vi "check Channel to read.vi"() -> ()   [LabVIEW 2019]
uses:
  Controls/Station - Test Type.ctl
  Controls/Global - Device.vi
  Controls/Global - IP Address.vi
  Controls/Global - Device Type.vi
panel:
  out "Array":i32[](array[numeric])
  out "Control Device":i32[](array[numeric])
  out "Device ID":i32[](array[numeric])
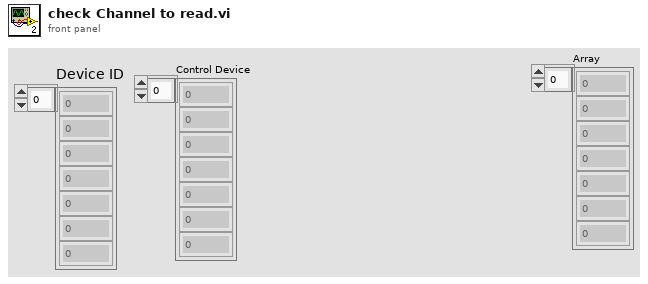
[diagram p1: front panel]
types:
  T1 = typedef "Station - Test Type.ctl" = u16
  T2 = cluster{"Station Name":string, "Key Value":string[], "Key Names":string[]}[]
  T3 = cluster{"Station Name":string, "Key Value":string[], "Key Names":string[]}
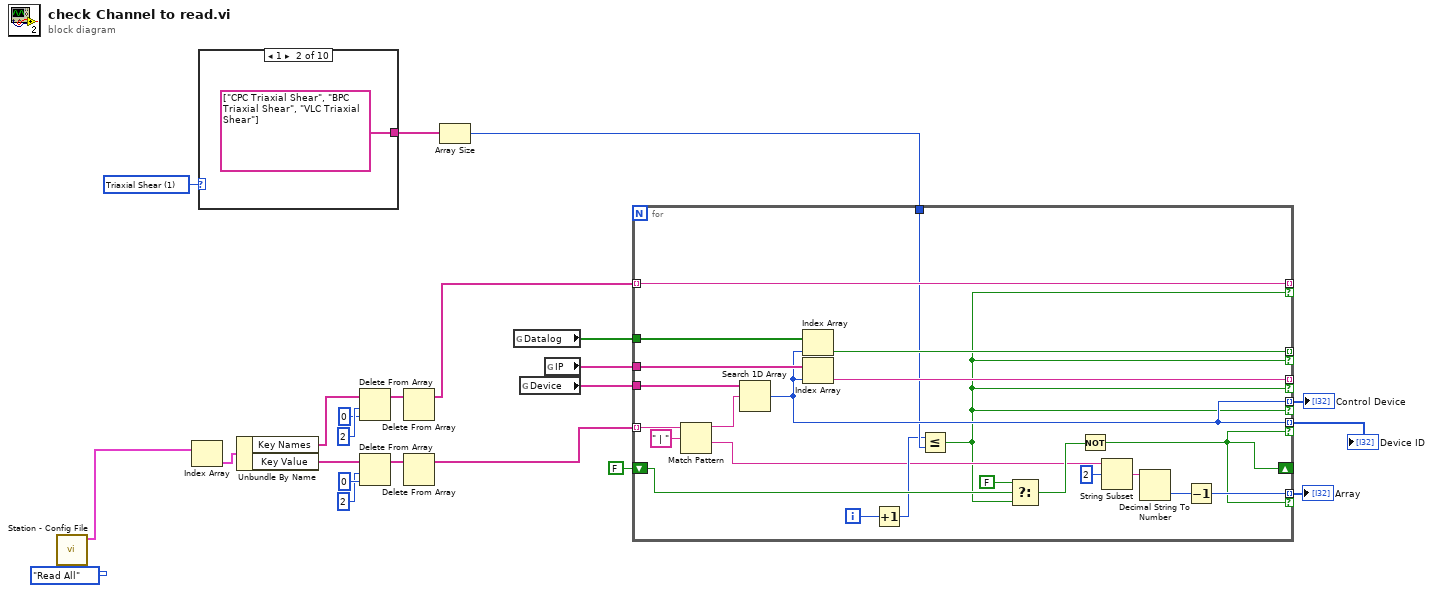
[diagram p0: block diagram]
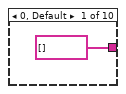
[diagram p2: hidden frame]
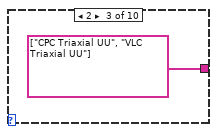
[diagram p3: hidden frame]
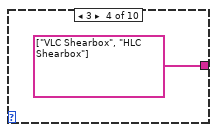
[diagram p4: hidden frame]
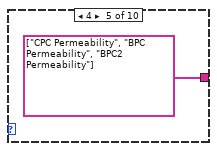
[diagram p5: hidden frame]
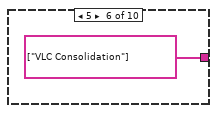
[diagram p6: hidden frame]
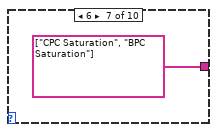
[diagram p7: hidden frame]
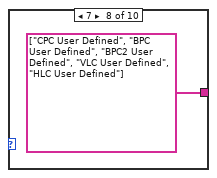
[diagram p8: hidden frame]
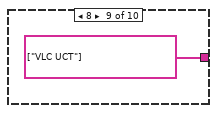
[diagram p9: hidden frame]
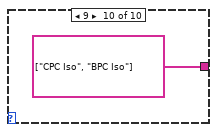
[diagram p10: hidden frame]
diagram:
  w3 = T1 1 items=["Please Select", "Triaxial Shear", "Triaxial UU", "Shearbox", "Permeability", "Consolidation (Stepped Loading)/Swelling", "Saturation (Incremental)", "User Defined", "UCT", "Isotropic Consolidation"] ("Test Type")
  n1 = call "Station - Config File.vi"("Action"=enum16{"Write", "Read", "Read All", "Remove"}."Read All") -> ("Value Out"=w17:T2)  [unwired: 9 in, 1 out]
  n2 = Index Array(array=w17) -> (element=w23:T3)  [unwired: 1 in]
  n3 = case shown="1" w3 {
    tunnel: [string[] [] string[] ["CPC Triaxial Shear", "BPC Triaxial Shear", "VLC Triaxial Shear"] string[] ["CPC Triaxial UU", "VLC Triaxial UU"] string[] ["VLC Shearbox", "HLC Shearbox"] string[] ["CPC Permeability", "BPC Permeability", "BPC2 Permeability"] string[] ["VLC Consolidation"] string[] ["CPC Saturation", "BPC Saturation"] string[] ["CPC User Defined", "BPC User Defined", "BPC2 User Defined", "VLC User Defined", "HLC User Defined"] string[] ["VLC UCT"] string[] ["CPC Iso", "BPC Iso"]] -> w4
    frame 0, Default {
    }
    frame 1 {
    }
    frame 2 {
    }
    frame 3 {
    }
    frame 4 {
    }
    frame 5 {
    }
    frame 6 {
    }
    frame 7 {
    }
    frame 8 {
    }
    frame 9 {
    }
  }
  n4 = Unbundle By Name(w23) -> ("Key Names"=w7:string[], "Key Value"=w22:string[])
  n5 = Delete From Array(array=w7, length=2, index=0) -> (array with subset deleted=w6:string[])  [unwired: 1 out]
  n6 = Delete From Array(array=w22, length=2, index=0) -> (array with subset deleted=w20:string[])  [unwired: 1 out]
  n7 = Delete From Array(array=w6) -> (array with subset deleted=w5:string[])  [unwired: 2 in, 1 out]
  n8 = Delete From Array(array=w20) -> (array with subset deleted=w16:string[])  [unwired: 2 in, 1 out]
  n9 = Array Size(array=w4) -> (size(s)=w2:i32)
  n10 = global read "Global - Device Type.vi" "Datalog"() -> (w10:bool[])
  n11 = global read "Global - Device.vi" "Device"() -> (w15:string[])
  n12 = global read "Global - IP Address.vi" "IP"() -> (w11:string[])
  n13 = for {
    tunnel: w16 -> [w55] mode=indexing
    tunnel: [w51] -> w1 mode=indexing if=w48
    tunnel: w15 -> [w50]
    tunnel: [w42] -> w14 mode=indexing if=w48
    shift-right: [w48] -> _
    shift-left: FALSE -> [w47]
    tunnel: [w42] -> w12 mode=indexing if=w34
    tunnel: w11 -> [w44]
    tunnel: [w43] -> _ mode=indexing if=w34
    tunnel: w10 -> [w41]
    tunnel: [w40] -> _ mode=indexing if=w34
    tunnel: w5 -> [w39] mode=indexing
    tunnel: [w39] -> _ mode=indexing if=w34
    tunnel: w2 -> [w37]
    i -> [w38]
    n14 = Match Pattern(string=w55, regular expression=" | ") -> (before substring=w49:string, after substring=w35:string)  [unwired: 1 in, 2 out]
    n15 = Search 1D Array(1D array=w50, element=w49) -> (index of element=w42:i32)  [unwired: 1 in]
    n16 = Index Array(array=w41, index=w42) -> (element=w40:bool)
    n17 = Index Array(array=w44, index=w42) -> (element=w43:string)
    n18 = Increment(x=w38) -> (x+1=w36:i32)
    n19 = Less Or Equal?(x=w36, y=w37) -> (x <= y?=w34:bool)
    n20 = Select(t=FALSE, s=w47, f=w34) -> (s? t:f=w46:bool)
    n21 = Not(x=w46) -> (.not. x?=w48:bool)
    n22 = String Subset(string=w35, offset (0)=2) -> (substring=w54:string)  [unwired: 1 in]
    n23 = Decimal String To Number(string=w54) -> (number=w52:i32)  [unwired: 2 in, 1 out]
    n24 = Decrement(x=w52) -> (x-1=w51:i32)
  }
  "Device ID" <- w14
  "Control Device" <- w12
  "Array" <- w1
